vi "Evaluate Transitions and Dwell Limits.vi"(1 "Boolean State Data in":T1, 2 "Stage Dwell Limit":u16, 3 "Event Dwell Limit":u16) -> (0 "Boolean State Data out":T1)   [LabVIEW 2015]
uses:
  Types/Injection Capture Core Boolean State Data.ctl
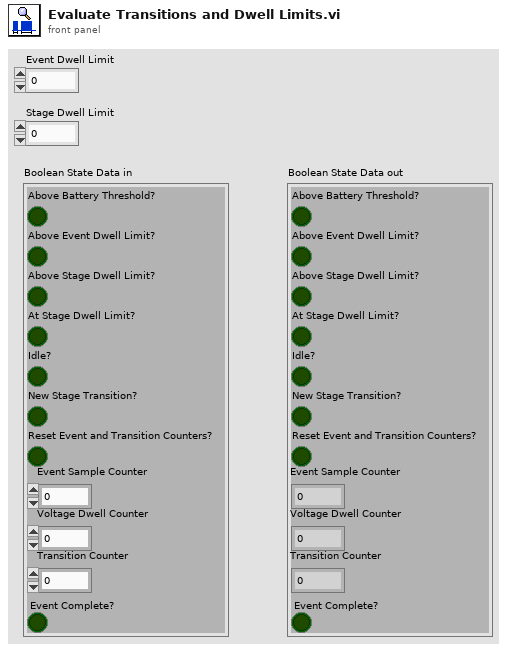
[diagram p1: front panel]
types:
  T1 = typedef "Injection Capture Core Boolean State Data.ctl" = cluster{"Above Battery Threshold?":bool, "Above Event Dwell Limit?":bool, "Above Stage Dwell Limit?":bool, "At Stage Dwell Limit?":bool, "Idle?":bool, "New Stage Transition?":bool, "Reset Event and Transition Counters?":bool, "Event Sample Counter":u16, "Voltage Dwell Counter":u32, "Transition Counter":u8, "Event Complete?":bool}
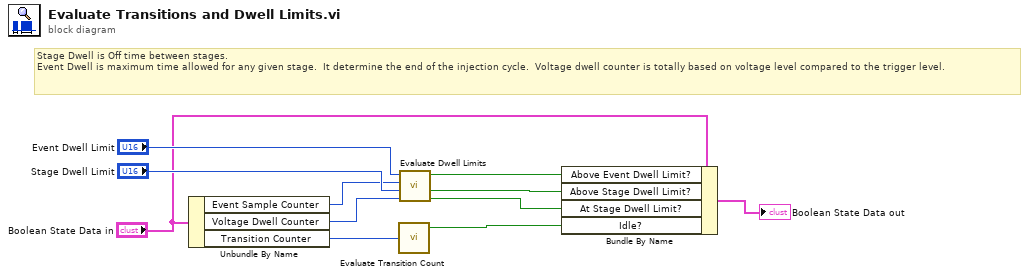
[diagram p0: block diagram]
diagram:
  # "Stage Dwell is Off time between stages.\nEvent Dwell is maximum time allowed for any given stage.  It determine the end of the injection cycle.  Voltage dwell counter is totally based on voltage level compared to the trigger level."
  n1 = Unbundle By Name("Boolean State Data in") -> ("Event Sample Counter"=w1:u16, "Voltage Dwell Counter"=w4:u32, "Transition Counter"=w3:u8)
  n2 = call "Evaluate Transition Count.vi"("Transition Count"=w3) -> ("Idle?"=w6:bool)  [unwired: 4 in]
  n3 = call "Evaluate Dwell Limits.vi"("Voltage Dwell Count"=w4, "Stage Dwell Limit"="Stage Dwell Limit", "Event Count"=w1, "Event Dwell Limit"="Event Dwell Limit") -> ("At Stage Dwell Limit?"=w7:bool, "Above Stage Dwell Limit?"=w8:bool, "Above Event Dwell Limit?"=w9:bool)  [unwired: 5 in]
  n4 = Bundle By Name(cluster="Boolean State Data in", "Above Event Dwell Limit?"=w9, "Above Stage Dwell Limit?"=w8, "At Stage Dwell Limit?"=w7, "Idle?"=w6) -> (→"Boolean State Data out":T1)
